vi "DAQmx Create Channel (DO-Digital Output).vi"(0 "task in":refnum<k21>, 5 "lines":tag, 7 "name to assign":string, 9 "line grouping":i32(ring)=1 items=["one channel for each line", "one channel for all lines"], 11 "error in":errorcluster) -> (4 "task out":refnum<k21>, 15 "error out":errorcluster)   [LabVIEW 2020]
doc: "Creates channel(s) to generate digital signals. You can group digital lines into one digital channel or separate them into multiple digital channels. If you specify one or more entire ports in <B>lines</B> input by using port physical channel names, you cannot separate the ports into multiple channels. To separate ports into multiple channels, use this VI multiple times with a different port each time."
uses:
  nilvaiu.dll
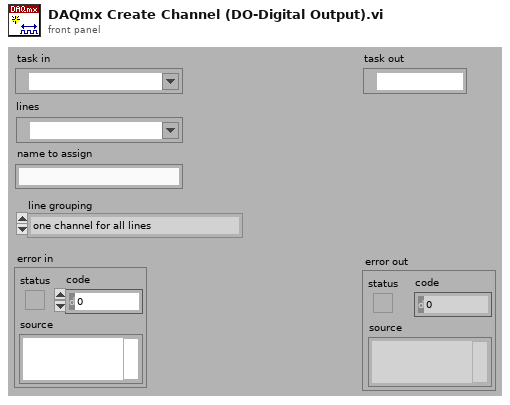
[diagram p1: front panel]
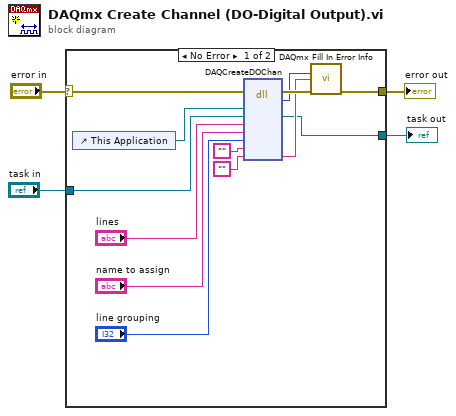
[diagram p0: block diagram]
diagram:
  n1 = case shown="No Error" "error in" {
    selector: "error in" -> [w6 w19]
    tunnel: [w12 w19] -> w4
    tunnel: "task in" -> [w8 w18]
    tunnel: [w7 w18] -> w2
    frame No Error {
      n2 = control-ref of="This Application"() -> (w17:refnum<vi>)
      n3 = dll-call lib="nilvaiu.*" fn="DAQCreateDOChan"(error in=w6, "lvAppRef"=w17, "refObjPtr"=w8, "lines"="lines", "channelNameIn"="name to assign", "lineGrouping"="line grouping", "channelNamesOut"="", "extendedErrorInfo"="") -> (error out=w15:errorcluster, "return type"=w13:i32, "refObjPtr"=w7:refnum<k21>, "extendedErrorInfo"=w14:string)  [unwired: 7 in, 1 out]
      n4 = call "DAQmx Fill In Error Info.vi"("status code"=w13, "extended error info"=w14, "error in"=w15) -> ("error out"=w12:errorcluster)  [unwired: 1 in, 11 out]
    }
    frame Error {
    }
  }
  "error out" <- w4
  "task out" <- w2
